vi "gun_map_mode_to_preset.vi"(11 "gun tracking mode":T2) -> (3 "Preset Position":T1)   [LabVIEW 2011]
uses:
  gun_tracking_mode.ctl
  gun_preset_pos_t.ctl
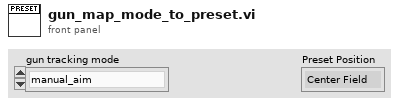
[diagram p1: front panel]
types:
  T1 = typedef "gun_preset_pos_t.ctl" = enum16{"Center Field", "Right Pocket", "Left Pocket", "Align Center", "Align Center Backwards", "Fold Side", "Pass"}
  T2 = typedef "gun_tracking_mode.ctl" = enum16{"manual_aim", "auto_aim_camera", "preset_center_field", "preset_right_pocket", "preset_left_pocket", "align_center", "align_center_backwards", "auto_aim_key", "align_fold", "auton_custom", "preset_pass", "auto_aim_auton"}
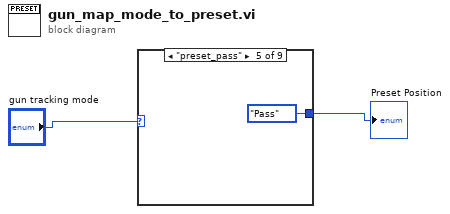
[diagram p0: block diagram]
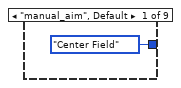
[diagram p2: hidden frame]
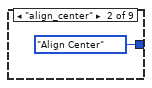
[diagram p3: hidden frame]
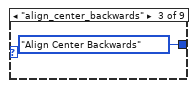
[diagram p4: hidden frame]
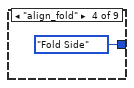
[diagram p5: hidden frame]
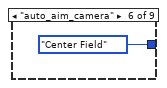
[diagram p6: hidden frame]
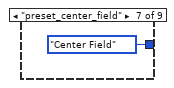
[diagram p7: hidden frame]
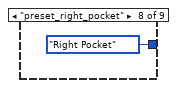
[diagram p8: hidden frame]
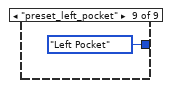
[diagram p9: hidden frame]
diagram:
  n1 = case shown="\"preset_pass\"" "gun tracking mode" {
    tunnel: [gun_preset_pos_t."Center Field" ("Preset Position") gun_preset_pos_t."Align Center" ("Preset Position") gun_preset_pos_t."Align Center Backwards" ("Preset Position") gun_preset_pos_t."Fold Side" ("Preset Position") gun_preset_pos_t."Pass" ("Preset Position") gun_preset_pos_t."Center Field" ("Preset Position") gun_preset_pos_t."Center Field" ("Preset Position") gun_preset_pos_t."Right Pocket" ("Preset Position") gun_preset_pos_t."Left Pocket" ("Preset Position")] -> w1
    frame "manual_aim", Default {
    }
    frame "align_center" {
    }
    frame "align_center_backwards" {
    }
    frame "align_fold" {
    }
    frame "preset_pass" {
    }
    frame "auto_aim_camera" {
    }
    frame "preset_center_field" {
    }
    frame "preset_right_pocket" {
    }
    frame "preset_left_pocket" {
    }
  }
  "Preset Position" <- w1
